vi "GetParentQualifiedName.vi"(8 "error in (no error)":errorcluster, 11 "ILabVIEWItem in":refnum<class "ILabVIEWItem.lvclass">) -> (0 "error out":errorcluster, 1 "Name":string, 3 "ILabVIEWItem out":refnum<class "ILabVIEWItem.lvclass">)   [LabVIEW 2020, in "LabVIEWObjectInterfaces.lvlib" / "ILabVIEWItem.lvclass"]
uses:
  ILabVIEWItem.lvclass
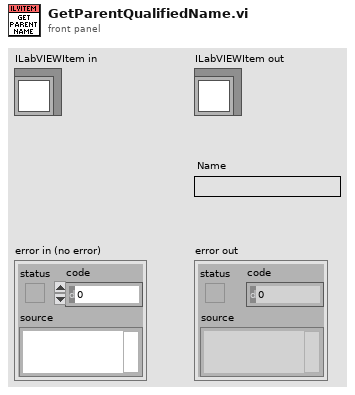
[diagram p1: front panel]
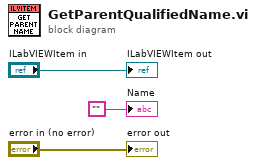
[diagram p0: block diagram]
diagram:
  "error out" <- "error in (no error)"
  "ILabVIEWItem out" <- "ILabVIEWItem in"
  "Name" <- ""
